vi "GetSchedule.vi"() -> ()   [LabVIEW 2018]
uses:
  <vilib>/Utility/config.llb/Write Key (I32).vi
  <vilib>/Utility/config.llb/NI_LVConfig.lvlib
panel:
  in  "Event":string="2018code"
  out "Team Matches info":T1(array[cluster])
  in  "Team#":i32=4153
  out "Matches data":string[][](array[string])
  out "innerText":string
  in  "WebBrowser":refnum<k7>(container)
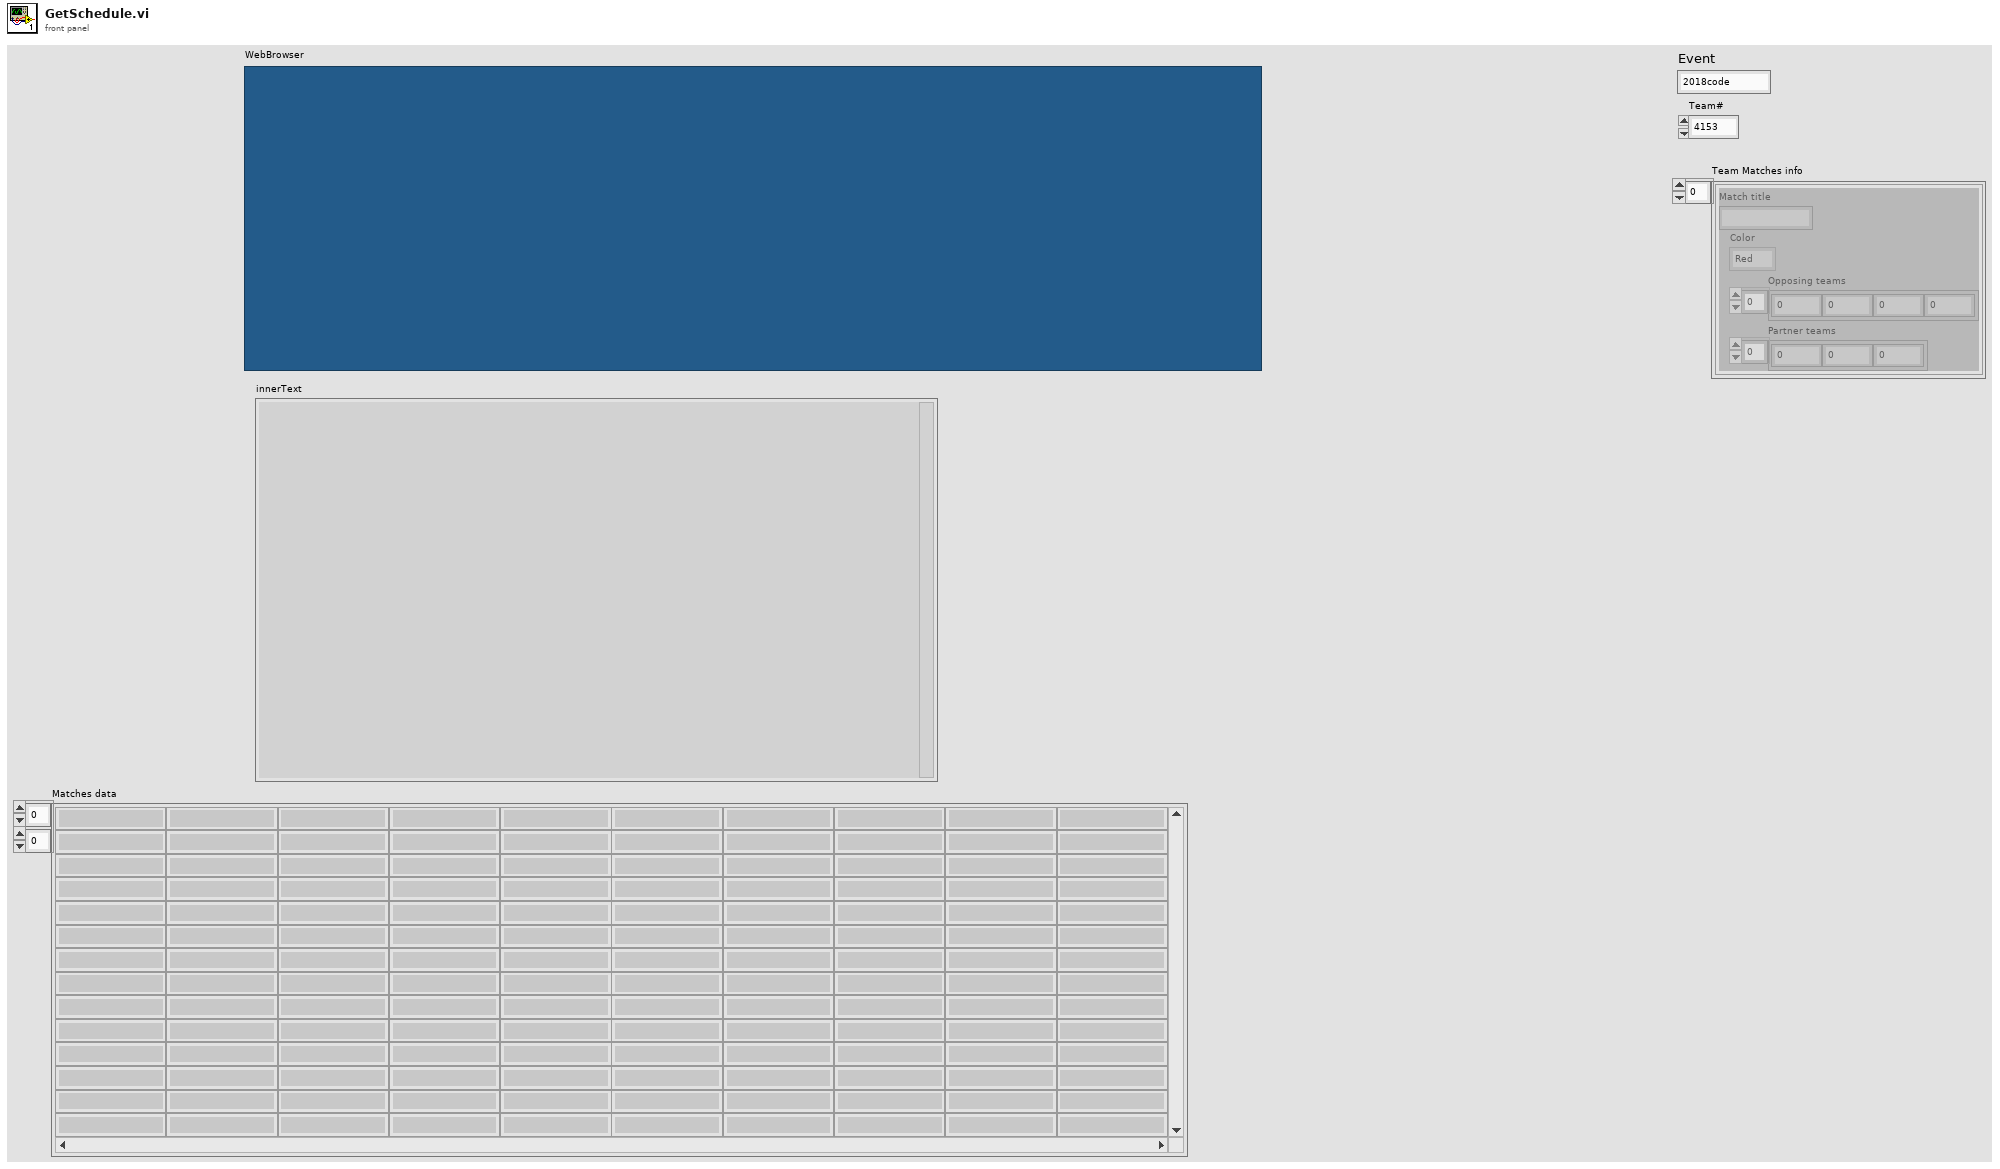
[diagram p1: front panel]
types:
  T1 = cluster{"Match title":string, "Color":enum16{"Red", "Blue"}, "Opposing teams":i32[], "Partner teams":i32[]}[]
  T2 = typedef "NI_LVConfig.lvlib/Config Data RefNum.ctl" = refnum<k1>
  T3 = cluster{"Match title":string, "Color":enum16{"Red", "Blue"}, "Opposing teams":i32[], "Partner teams":i32[]}
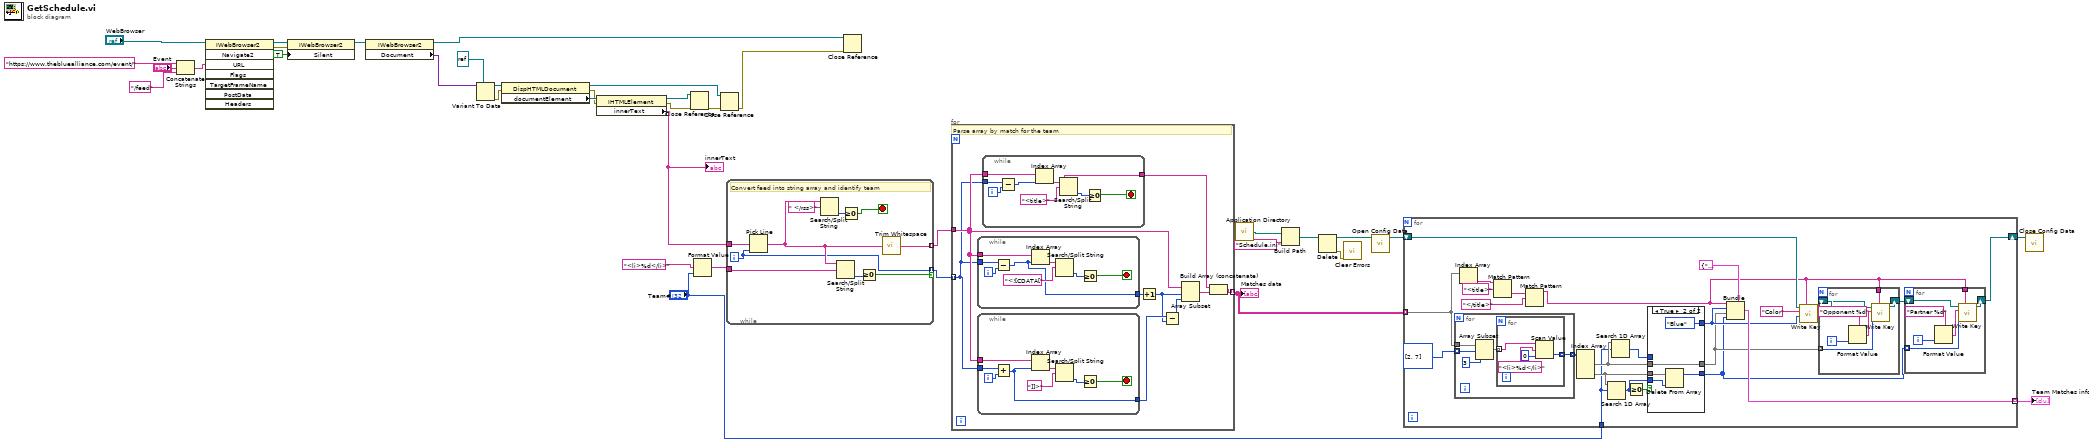
[diagram p0: block diagram]
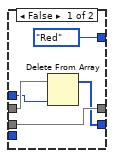
[diagram p2: hidden frame]
diagram:
  n1 = Concatenate Strings("https://www.thebluealliance.com/event/", "Event", "/feed" ("string")) -> (w2:string)
  n2 = invoke class="IWebBrowser2" method="Navigate2"(reference="WebBrowser", "URL"=w2) -> (reference out=w36:refnum<k7>, error out=w34:errorcluster)  [unwired: 6 in, 6 out]
  n3 = property class="IWebBrowser2"(reference=w36, error in=w34, "Silent"=TRUE) -> (reference out=w33:refnum<k7>)  [unwired: 1 out]
  n4 = property class="IWebBrowser2"(reference=w33) -> (reference out=w31:refnum<k7>, "Document"=w25:variant)  [unwired: 1 in, 1 out]
  n5 = Variant To Data(type=refnum<k7> refnum ("reference out"), Variant=w25) -> (data=w30:refnum<k7>, error out=w27:errorcluster)  [unwired: 1 in]
  n6 = property class="DispHTMLDocument"(reference=w30, error in=w27) -> (reference out=w21:refnum<k7>, error out=w26:errorcluster, "documentElement"=w28:refnum<k7>)
  n7 = property class="IHTMLElement"(reference=w28, error in=w26) -> (reference out=w23:refnum<k7>, error out=w24:errorcluster, "innerText"=w17:string)
  "innerText" <- w17
  n8 = Close Reference(reference=w23, error in (no error)=w24) -> (error out=w22:errorcluster)
  n9 = Format Value(format string="<li>%d</li>" ("string (\"\")"), value (0)="Team#") -> (output string=w18:string)  [unwired: 1 in]
  n10 = Close Reference(reference=w21, error in (no error)=w22) -> (error out=w20:errorcluster)
  n11 = while {
    tunnel: w17 -> [w46]
    tunnel: w18 -> [w40]
    tunnel: [w42] -> w15 mode=indexing
    tunnel: [w38] -> w16 mode=indexing if=w37
    i -> [w38]
    stop <- w43 stop-if-true
    # "Convert feed into string array and identify team"
    n12 = Pick Line(multi-line string=w46, line index=w38) -> (output string=w41:string)  [unwired: 1 in]
    n13 = Search/Split String(string=w41, search string/char (-)=" </rss>") -> (offset of match=w44:i32)  [unwired: 1 in, 2 out]
    n14 = Search/Split String(string=w41, search string/char (-)=w40) -> (offset of match=w39:i32)  [unwired: 1 in, 2 out]
    n15 = Greater Or Equal To 0?(x=w44) -> (x >= 0?=w43:bool)
    n16 = Greater Or Equal To 0?(x=w39) -> (x >= 0?=w37:bool)
    n17 = call <vilib>:"Trim Whitespace.vi"("string"=w41) -> ("trimmed string"=w42:string)  [unwired: 1 in]
  }
  n18 = Close Reference(reference=w31, error in (no error)=w20) -> ()  [unwired: 1 out]
  n19 = for {
    tunnel: w16 -> [w49] mode=indexing
    tunnel: w15 -> [w50]
    tunnel: [w48] -> w14 mode=indexing
    # "Parse array by match for the team"
    n20 = while {
      tunnel: w50 -> [w79]
      tunnel: w49 -> [w78]
      tunnel: [w72] -> w52
      i -> [w73]
      stop <- w75 stop-if-true
      n21 = Subtract(x=w78, y=w73) -> (x-y=w72:i32)
      n22 = Index Array(array=w79, index=w72) -> (element=w77:string)
      n23 = Search/Split String(string=w77, search string/char (-)="<![CDATA[") -> (offset of match=w76:i32)  [unwired: 1 in, 2 out]
      n24 = Greater Or Equal To 0?(x=w76) -> (x >= 0?=w75:bool)
    }
    n25 = while {
      tunnel: w50 -> [w71]
      tunnel: w49 -> [w70]
      tunnel: [w64] -> w54
      i -> [w65]
      stop <- w67 stop-if-true
      n26 = Add(x=w70, y=w65) -> (x+y=w64:i32)
      n27 = Index Array(array=w71, index=w64) -> (element=w69:string)
      n28 = Search/Split String(string=w69, search string/char (-)="]]>") -> (offset of match=w68:i32)  [unwired: 1 in, 2 out]
      n29 = Greater Or Equal To 0?(x=w68) -> (x >= 0?=w67:bool)
    }
    n30 = while {
      tunnel: w50 -> [w63]
      tunnel: w49 -> [w62]
      tunnel: [w56] -> w47
      i -> [w58]
      stop <- w60 stop-if-true
      n31 = Subtract(x=w62, y=w58) -> (x-y=w57:i32)
      n32 = Index Array(array=w63, index=w57) -> (element=w56:string)
      n33 = Search/Split String(string=w56, search string/char (-)="<title>") -> (offset of match=w61:i32)  [unwired: 1 in, 2 out]
      n34 = Greater Or Equal To 0?(x=w61) -> (x >= 0?=w60:bool)
    }
    n35 = Increment(x=w52) -> (x+1=w51:i32)
    n36 = Subtract(x=w54, y=w51) -> (x-y=w55:i32)
    n37 = Array Subset(array=w50, index=w51, length=w55) -> (w53:string[])
    n38 = Build Array (concatenate)(w47, w53) -> (w48:string[])
  }
  "Matches data" <- w14
  n39 = call <vilib>:"Application Directory.vi"() -> ("Application Directory"=w11:path)
  n40 = Build Path(base path=w11, name or relative path="Schedule.ini") -> (appended path=w9:path)
  n41 = Delete(path (use dialog)=w9) -> (deleted path=w6:path, error out=w5:errorcluster)  [unwired: 4 in, 1 out]
  n42 = call <vilib>:"Clear Errors.vi"("error in (no error)"=w5) -> ()  [unwired: 5 in, 2 out]
  n43 = call <vilib>:"Open Config Data.vi"("configuration file path"=w6) -> ("refnum"=w8:T2)  [unwired: 8 in, 2 out]
  n44 = for {
    tunnel: w14 -> [w97] mode=indexing
    tunnel: [w98] -> w12 mode=indexing
    tunnel: "Team#" -> [w89]
    shift-right: [w82] -> w7
    shift-left: w8 -> [w88]
    n45 = for {
      tunnel: w97 -> [w132]
      tunnel: [w129] -> w96 mode=indexing
      tunnel: i32[] [2, 7] ("index") -> [w128] mode=indexing
      n46 = Array Subset(array=w132, index=w128, length=3 ("index")) -> (w130:string[])
      n47 = for {
        tunnel: w130 -> [w135] mode=indexing
        tunnel: [w133] -> w129 mode=indexing
        n48 = Scan Value(string=w135, format string="<li>%d</li>" ("string (\"\")"), default (0 dbl)=0 ("Opposing teams")) -> (value=w133:i32)  [unwired: 1 out]
      }
    }
    n49 = Index Array(array=w97) -> (element=w101:string)  [unwired: 1 in]
    n50 = Match Pattern(string=w101, regular expression="<title>" ("search string/char (-)")) -> (after substring=w100:string)  [unwired: 1 in, 3 out]
    n51 = Match Pattern(string=w100, regular expression="</title>" ("search string/char (-)")) -> (before substring=w81:string)  [unwired: 1 in, 3 out]
    n52 = Index Array(array=w96) -> (element #1=w91:i32[], element #2=w94:i32[])  [unwired: 4 in]
    n53 = Search 1D Array(1D array=w94, element=w89) -> (index of element=w92:i32)  [unwired: 1 in]
    n54 = Search 1D Array(1D array=w91, element=w89) -> (index of element=w90:i32)  [unwired: 1 in]
    n55 = Greater Or Equal To 0?(x=w92) -> (x >= 0?=w93:bool)
    n56 = case shown="True" w93 {
      tunnel: w91 -> [w122 w127]
      tunnel: [w120 w127] -> w84
      tunnel: [w119 w125] -> w80
      tunnel: w94 -> [w120 w126]
      tunnel: w92 -> [_ w124]
      tunnel: w90 -> [w121 _]
      tunnel: [enum16{"Red", "Blue"}."Red" ("Color") enum16{"Red", "Blue"}."Blue" ("Color")] -> w86
      frame False {
        n57 = Delete From Array(array=w122, index=w121) -> (array with subset deleted=w119:i32[])  [unwired: 1 in, 1 out]
      }
      frame True {
        n58 = Delete From Array(array=w126, index=w124) -> (array with subset deleted=w125:i32[])  [unwired: 1 in, 1 out]
      }
    }
    n59 = Bundle(cluster=T3 {"Match title"="", "Color"=enum."Blue", "Opposing teams"=[], "Partner teams"=[]}, "Match title"=w81, "Color"=w86, "Opposing teams"=w84, "Partner teams"=w80) -> (w98:T3)
    n60 = call-poly <vilib>:"Write Key.vi"("section"=w81, "value"=w86, "key"="Color", "refnum"=w88) -> ("refnum out"=w85:T2)  [unwired: 5 in, 2 out]
    n61 = for {
      tunnel: w81 -> [w115]
      shift-right: [w114] -> w83
      shift-left: w85 -> [w116]
      tunnel: w84 -> [w111] mode=indexing
      i -> [w112]
      n62 = Format Value(format string="Opponent %d" ("key"), value (0)=w112) -> (output string=w113:string)  [unwired: 1 in]
      n63 = call-poly <vilib>:"Write Key.vi"("section"=w115, "value"=w111, "key"=w113, "refnum"=w116) -> ("refnum out"=w114:T2)  [unwired: 5 in, 2 out]
    }
    n64 = for {
      tunnel: w81 -> [w108]
      shift-right: [w107] -> w82
      shift-left: w83 -> [w109]
      tunnel: w80 -> [w104] mode=indexing
      i -> [w105]
      n65 = Format Value(format string="Partner %d" ("key"), value (0)=w105) -> (output string=w106:string)  [unwired: 1 in]
      n66 = call-poly <vilib>:"Write Key.vi"("section"=w108, "value"=w104, "key"=w106, "refnum"=w109) -> ("refnum out"=w107:T2)  [unwired: 5 in, 2 out]
    }
  }
  "Team Matches info" <- w12
  n67 = call <vilib>:"Close Config Data.vi"("refnum"=w7) -> ()  [unwired: 9 in, 2 out]
